vi "Get Needed Points.vi"(8 "error in (no error)":errorcluster, 11 "Tool Path in":refnum<class "Tool Path.lvclass">) -> (0 "error out":errorcluster, 3 "Tool Path out":refnum<class "Tool Path.lvclass">)   [LabVIEW 2019, in "Tool Path.lvclass"]
uses:
  Tool Path.lvclass
  Parse/ParsePaths/Path.lvclass/Path.ctl
  Parse/PathCommands/PathCommands.lvclass
  Parse/ParsePaths/Path.lvclass
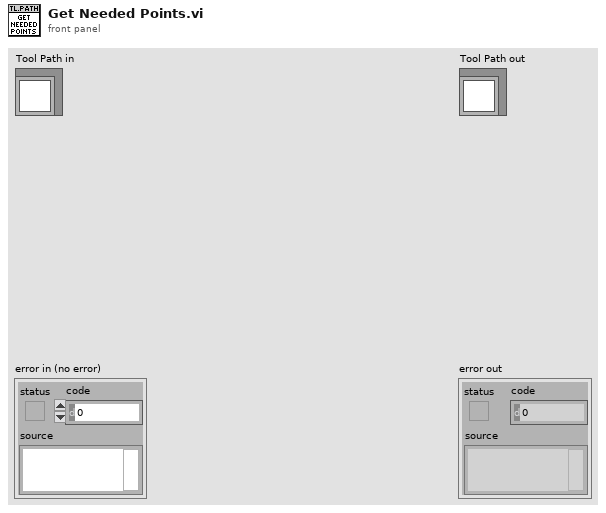
[diagram p1: front panel]
types:
  T1 = enum16{"None", "After", "Before", "Last", "First"}[]
  T2 = typedef "PathCommands.lvclass/Point.ctl" = cluster{"X":dbl, "Y":dbl}
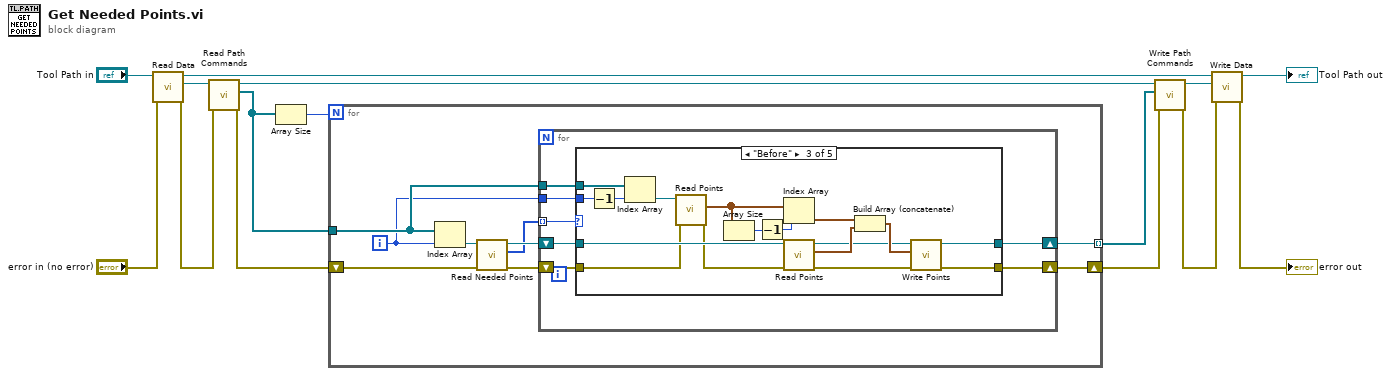
[diagram p0: block diagram]
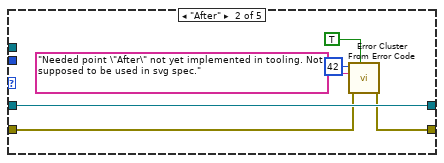
[diagram p3: hidden frame]
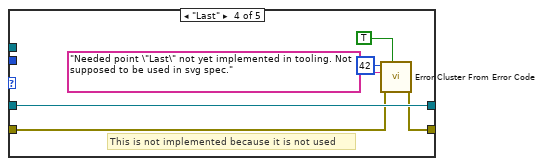
[diagram p4: hidden frame]
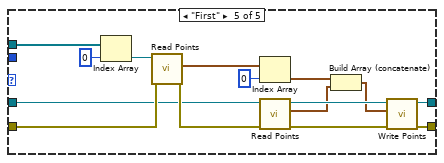
[diagram p5: hidden frame]
diagram:
  n1 = call-dynamic "Read Data.vi"("error in (no error)"="error in (no error)", "Tool Path in"="Tool Path in") -> ("error out"=w4:errorcluster, "Path.lvclass"=w9:refnum<class "Path.lvclass">, "Tool Path out"=w7:refnum<class "Tool Path.lvclass">)  [unwired: 7 in]
  n2 = call "Read Path Commands.vi"("error in (no error)"=w4, "Path in"=w9) -> ("error out"=w11:errorcluster, "Path Commands"=w14:refnum<class "PathCommands.lvclass">[], "Path out"=w13:refnum<class "Path.lvclass">)  [unwired: 7 in]
  n3 = Array Size(array=w14) -> (size(s)=w15:i32)
  n4 = for {
    N: w15 -> [_]
    tunnel: w14 -> [w19]
    shift-right: [w17] -> w10
    shift-left: w11 -> [w24]
    tunnel: [w16] -> w12 mode=indexing
    i -> [w18]
    n5 = Index Array(array=w19, index=w18) -> (element=w23:refnum<class "PathCommands.lvclass">)
    n6 = call-dynamic "Read Needed Points.vi"("error in (no error)"=w24, "PathCommands in"=w23) -> ("error out"=w22:errorcluster, "Needed Points"=w20:T1, "PathCommands out"=w21:refnum<class "PathCommands.lvclass">)  [unwired: 7 in]
    n7 = for {
      shift-right: [w29] -> w16
      shift-left: w21 -> [w28]
      shift-right: [w30] -> w17
      shift-left: w22 -> [w31]
      tunnel: w20 -> [w27] mode=indexing
      tunnel: w19 -> [w26]
      tunnel: w18 -> [w25]
      n8 = case shown="\"Before\"" w27 {
        tunnel: w31 -> [w33 w34 w48 w60 w69]
        tunnel: [w33 w35 w41 w61 w68] -> w30
        tunnel: [w32 w39 w43 w62 w67] -> w29
        tunnel: w28 -> [w32 w39 w49 w62 w66]
        tunnel: w26 -> [_ _ w56 _ w64]
        tunnel: w25 -> [_ _ w54 _ _]
        frame "None", Default {
        }
        frame "After" {
          n9 = call <vilib>:"Error Cluster From Error Code.vi"("show call chain? (False)"=TRUE, "error in (no error)"=w34, "error message (\"\")"="Needed point \"After\" not yet implemented in tooling. Not supposed to be used in svg spec." ("error message (\"\")"), "error code (0)"=42) -> ("error out"=w35:errorcluster)  [unwired: 5 in]
        }
        frame "Before" {
          n10 = Decrement(x=w54) -> (x-1=w55:i32)
          n11 = Index Array(array=w56, index=w55) -> (element=w53:refnum<class "PathCommands.lvclass">)
          n12 = call-dynamic "Read Points.vi"("error in (no error)"=w48, "PathCommands in"=w53) -> ("error out"=w47:errorcluster, "Points"=w52:T2[])  [unwired: 7 in, 1 out]
          n13 = Array Size(array=w52) -> (size(s)=w51:i32)
          n14 = Decrement(x=w51) -> (x-1=w50:i32)
          n15 = Index Array(array=w52, index=w50) -> (element=w46:T2)
          n16 = call-dynamic "Read Points.vi"("error in (no error)"=w47, "PathCommands in"=w49) -> ("error out"=w40:errorcluster, "Points"=w45:T2[], "PathCommands out"=w42:refnum<class "PathCommands.lvclass">)  [unwired: 7 in]
          n17 = Build Array (concatenate)(w46, w45) -> (w44:T2[])
          n18 = call-dynamic "Write Points.vi"("error in (no error)"=w40, "Points"=w44, "PathCommands in"=w42) -> ("error out"=w41:errorcluster, "PathCommands out"=w43:refnum<class "PathCommands.lvclass">)  [unwired: 7 in]
        }
        frame "Last" {
          # "This is not implemented because it is not used"
          n19 = call <vilib>:"Error Cluster From Error Code.vi"("show call chain? (False)"=TRUE, "error in (no error)"=w60, "error message (\"\")"="Needed point \"Last\" not yet implemented in tooling. Not supposed to be used in svg spec." ("error message (\"\")"), "error code (0)"=42) -> ("error out"=w61:errorcluster)  [unwired: 5 in]
        }
        frame "First" {
          n20 = Index Array(array=w64, index=0) -> (element=w70:refnum<class "PathCommands.lvclass">)
          n21 = call-dynamic "Read Points.vi"("error in (no error)"=w69, "PathCommands in"=w70) -> ("error out"=w72:errorcluster, "Points"=w71:T2[])  [unwired: 7 in, 1 out]
          n22 = Index Array(array=w71, index=0) -> (element=w73:T2)
          n23 = call-dynamic "Read Points.vi"("error in (no error)"=w72, "PathCommands in"=w66) -> ("error out"=w77:errorcluster, "Points"=w74:T2[], "PathCommands out"=w76:refnum<class "PathCommands.lvclass">)  [unwired: 7 in]
          n24 = Build Array (concatenate)(w73, w74) -> (w75:T2[])
          n25 = call-dynamic "Write Points.vi"("error in (no error)"=w77, "Points"=w75, "PathCommands in"=w76) -> ("error out"=w68:errorcluster, "PathCommands out"=w67:refnum<class "PathCommands.lvclass">)  [unwired: 7 in]
        }
      }
    }
  }
  n26 = call "Write Path Commands.vi"("error in (no error)"=w10, "Path Commands"=w12, "Path in"=w13) -> ("error out"=w3:errorcluster, "Path out"=w8:refnum<class "Path.lvclass">)  [unwired: 7 in]
  n27 = call-dynamic "Write Data.vi"("error in (no error)"=w3, "Path.lvclass"=w8, "Tool Path in"=w7) -> ("error out"=→"error out":errorcluster, "Tool Path out"=→"Tool Path out":refnum<class "Tool Path.lvclass">)  [unwired: 7 in]
